vi "QTrkComputeLUTFisherMatrix.vi"(0 "LUT":sgl[][](array[numeric]), 5 "QTrk Settings":T3={"Image width"=150, "Image height"=150, "Number of threads (CPU based)"=-1, "CUDA Device"=-2, "COM Background correction factor"=0.0, "ZLUT MinRadius"=8.0, "ZLUT Radial Coverage"=5.0, "ZLUT Angular Coverage"=2.0, "ZLUT ROI Coverage"=0.7, "QI Iterations"=1, "QI MinRadius"=2.0, "QI Radial Coverage"=5.0, "QI Angular Coverage"=2.0, "QI ROI Coverage"=0.7, "QI Angular Step \nIteration Factor"=0.8, "XCOR Profile Length"=1, "XCOR Profile Width"=128, "XCOR Iterations"=32, "Gaussian 2D Fit Iterations"=2, "Gaussian 2D Sigma (pixels)"=3.0}, 7 "Initial variance estimate":T1, 9 "XYZ":T1, 11 "lutIntensityFactor":sgl=255.0, 12 "Nsamples":i32=20) -> (4 "XYZ Variance":T1, 6 "Fisher Matrix":T2, 10 "Inverse Fisher Matrix":T2)   [LabVIEW 2011]
uses:
  QTrkSettings.ctl
  XYZf.ctl
  <vilib>/Analysis/Matrix/Datatypes/RealMatrix.ctl
  QTrkDLL.vi
  <vilib>/Analysis/Matrix/Numeric/Conversions/Array To Matrix - RA2.vi
  <vilib>/Analysis/Matrix/NI_Matrix.lvlib
panel:
  # "-2: Use all devices\n-1: Use best device"
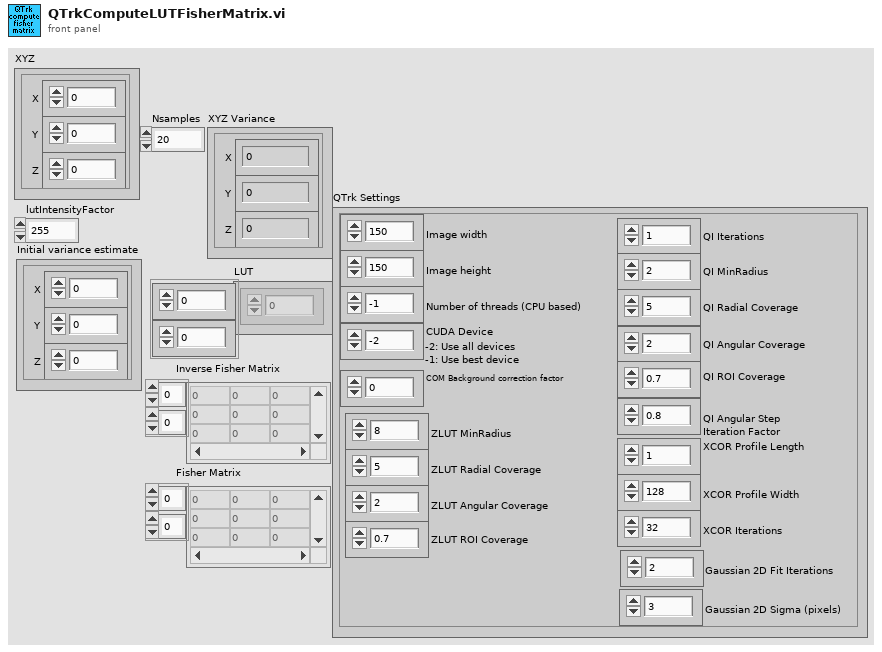
[diagram p1: front panel]
types:
  T1 = typedef "XYZf.ctl" = cluster{"X":sgl, "Y":sgl, "Z":sgl}
  T2 = typedef "NI_Matrix.lvlib/RealMatrix.ctl" = dbl[][]
  T3 = typedef "QTrkSettings.ctl" = cluster{"Image width":i32, "Image height":i32, "Number of threads (CPU based)":i32, "CUDA Device":i32, "COM Background correction factor":sgl, "ZLUT MinRadius":sgl, "ZLUT Radial Coverage":sgl, "ZLUT Angular Coverage":sgl, "ZLUT ROI Coverage":sgl, "QI Iterations":i32, "QI MinRadius":sgl, "QI Radial Coverage":sgl, "QI Angular Coverage":sgl, "QI ROI Coverage":sgl, "QI Angular Step \nIteration Factor":sgl, "XCOR Profile Length":i32, "XCOR Profile Width":i32, "XCOR Iterations":i32, "Gaussian 2D Fit Iterations":i32, "Gaussian 2D Sigma (pixels)":sgl}
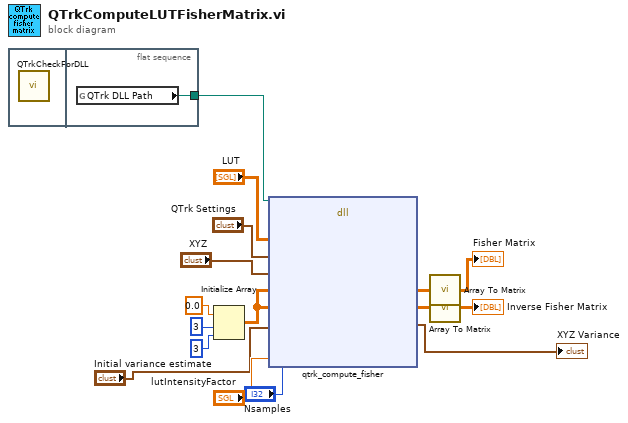
[diagram p0: block diagram]
diagram:
  n1 = flat-sequence {
    tunnel: [w17] -> w16
    frame #0 {
      n2 = call "QTrkCheckForDLL.vi"() -> ()  [unwired: 12 in]
    }
    frame #1 {
      n3 = global read "QTrkDLL.vi" "QTrk DLL Path"() -> (w17:path)
    }
  }
  n4 = Initialize Array(sgl 0.0 ("X"), 3 ("dimension size"), 3 ("dimension size")) -> (w11:sgl[][])
  n5 = dll-call lib="D:/jcnossen1/cudaqi-tracker/bin/jtrk-labview.dll" fn="qtrk_compute_fisher"(path in=w16, "lut"="LUT", "trackerSettings"="QTrk Settings", "position"="XYZ", "fisherMatrix"=w11, "inverseFisherMatrix"=w11, "xyzVariance"="Initial variance estimate", "Nsamples"="Nsamples", "lutIntensityFactor"="lutIntensityFactor") -> ("fisherMatrix"=w10:sgl[][], "inverseFisherMatrix"=w9:sgl[][], "xyzVariance"=→"XYZ Variance":T1)  [unwired: 8 in, 2 out]
  n6 = call-poly <vilib>:"Array To Matrix.vi"("Real 2D Array"=w10) -> ("Real Matrix"=→"Fisher Matrix":T2)
  n7 = call-poly <vilib>:"Array To Matrix.vi"("Real 2D Array"=w9) -> ("Real Matrix"=→"Inverse Fisher Matrix":T2)
